vi "AI Timestamp Precision.vi"() -> ()   [LabVIEW 2020]
uses:
  <vilib>/DAQmx/read.llb/DAQmx Read (Analog Wfm 1Chan NSamp).vi
  <vilib>/DAQmx/write.llb/DAQmx Write (Digital Bool 1Line 1Point).vi
  <vilib>/Utility/High Resolution Relative Seconds.vi
  Utility VIs/Controls/Utilities-Wait.vi/89bc9713-8f2c-40bd-a11f-1c800a437687.vi
  <vilib>/DAQmx/create/channels.llb/DAQmx Create Channel (DO-Digital Output).vi
  <vilib>/DAQmx/create/channels.llb/DAQmx Create Channel (AI-Voltage-Basic).vi
  <vilib>/DAQmx/configure/timing.llb/DAQmx Timing (Sample Clock).vi
  <vilib>/DAQmx/miscellaneous.llb/DAQmx Fill In Error Info.vi
  <vilib>/Utility/High Resolution Polling Wait.vi
panel:
  out "Iteration":i32
  out "Graph":waveform(dbl)(graph)
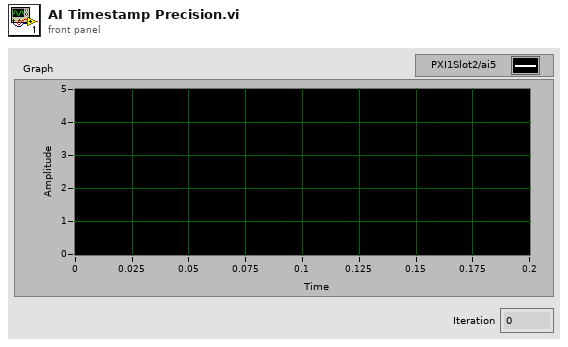
[diagram p1: front panel]
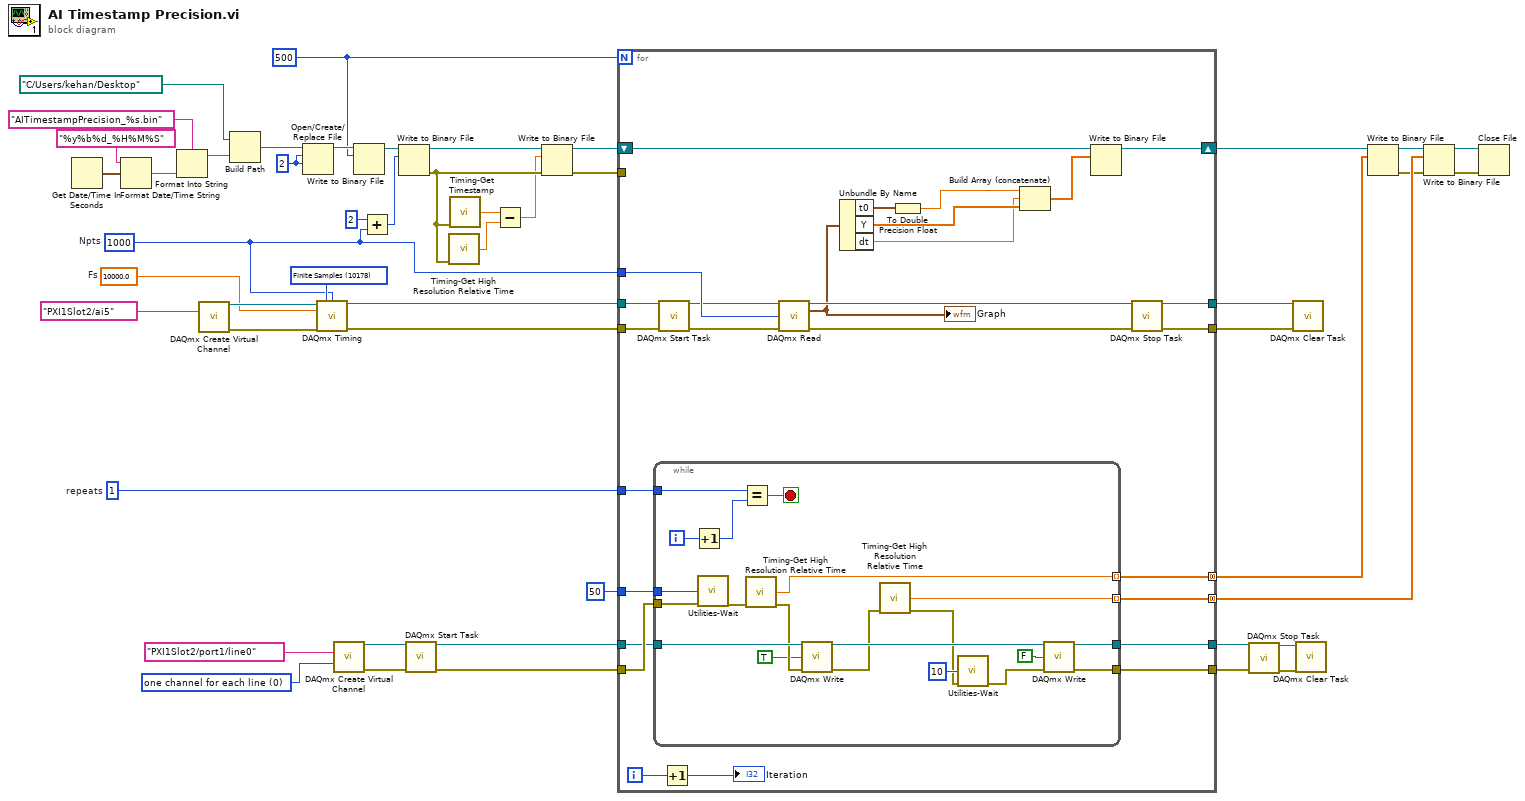
[diagram p0: block diagram]
diagram:
  w1 = 500
  w25 = u16 2
  w40 = 10000.0  # Fs
  w21 = 1000  # Npts
  w42 = 10178 items=["Finite Samples"=10178, "Continuous Samples"=10123, "Hardware Timed Single Point"=12522] ("sample mode")
  w22 = 1  # repeats
  w48 = 0 items=["one channel for each line", "one channel for all lines"] ("line grouping")
  n1 = Get Date/Time In Seconds() -> (seconds since 1Jan1904=w39:timestamp)
  n2 = Format Date/Time String(time format string (%c)="%y%b%d_%H%M%S", seconds (now)=w39) -> (date/time string=w37:string)  [unwired: 1 in]
  n3 = Format Into String(format string="AITimestampPrecision_%s.bin", w37) -> (resulting string=w34:string)  [unwired: 2 in, 1 out]
  n4 = call-poly <vilib>:"DAQmx Create Virtual Channel.vi"("physical channels"=tag "PXI1Slot2/ai5") -> ("task out"=w44:refnum<k21>, "error out"=w43:errorcluster)  [unwired: 13 in]
  n5 = Build Path(base path=path "C:/Users/kehan/Desktop" ("file path (use dialog)"), name or relative path=w34) -> (appended path=w33:path)
  n6 = Open/Create/Replace File(file path (use dialog)=w33, operation (0:open)=w25, access (0:read/write)=w25) -> (refnum out=w24:refnum<file>)  [unwired: 3 in, 2 out]
  n7 = call-poly <vilib>:"DAQmx Timing.vi"("task/channels in"=w44, "sample mode"=w42, "samples per channel"=w21, "rate"=w40, "error in"=w43) -> ("task out"=w11:refnum<k21>, "error out"=w10:errorcluster)  [unwired: 9 in]
  n8 = call-poly <vilib>:"DAQmx Create Virtual Channel.vi"("lines"=tag "PXI1Slot2/port1/line0", "line grouping"=w48) -> ("task out"=w46:refnum<k21>, "error out"=w45:errorcluster)  [unwired: 12 in]
  n9 = Write to Binary File(file (use dialog)=w24, data=w1) -> (refnum out=w23:refnum<file>)  [unwired: 4 in, 2 out]
  n10 = Add(x=2, y=w21) -> (x+y=w20:i32)
  n11 = Write to Binary File(file (use dialog)=w23, data=w20) -> (refnum out=w17:refnum<file>, error out=w16:errorcluster)  [unwired: 4 in, 1 out]
  n12 = call <vilib>:"DAQmx Start Task.vi"("task/channels in"=w46, "error in"=w45) -> ("task out"=w2:refnum<k21>, "error out"=w3:errorcluster)  [unwired: 12 in]
  n13 = call "Timing-Get High Resolution Relative Time.vi"("error in (no error)"=w16) -> ("double precision float"=w13:dbl)  [unwired: 13 in, 1 out]
  n14 = call "Timing-Get Timestamp.vi"("error in (no error)"=w16) -> ("double precision float"=w14:dbl)  [unwired: 13 in, 1 out]
  n15 = Subtract(x=w14, y=w13) -> (x-y=w12:dbl)
  n16 = Write to Binary File(file (use dialog)=w17, data=w12, error in=w16) -> (refnum out=w18:refnum<file>, error out=w15:errorcluster)  [unwired: 3 in, 1 out]
  n17 = for {
    N: w1 -> [_]
    tunnel: u32 50 ("milliseconds to wait") -> [w76]
    tunnel: [w71] -> w29 mode=concatenating
    tunnel: w22 -> [w70]
    tunnel: w21 -> [w69]
    tunnel: w15 -> [_]
    shift-right: [w73] -> w32
    shift-left: w18 -> [w68]
    tunnel: w11 -> [w61]
    tunnel: w10 -> [w60]
    tunnel: [w57] -> w9
    tunnel: [w56] -> w8
    tunnel: [w55] -> w7
    tunnel: [w54] -> w6
    tunnel: w3 -> [w53]
    tunnel: w2 -> [w52]
    tunnel: [w72] -> w31 mode=concatenating
    i -> [w51]
    n18 = while {
      tunnel: w52 -> [w96]
      tunnel: [w92] -> w55
      tunnel: [w91] -> w54
      tunnel: [w89] -> w71 mode=indexing
      tunnel: w70 -> [w90]
      tunnel: w76 -> [w88]
      tunnel: [w80] -> w72 mode=indexing
      tunnel: w53 -> [w77]
      i -> [w84]
      stop <- w85 stop-if-true
      n19 = Increment(x=w84) -> (x+1=w83:i32)
      n20 = call "Utilities-Wait.vi"("milliseconds to wait"=w88, "error in (no error)"=w77) -> ("error out"=w82:errorcluster)  [unwired: 13 in]
      n21 = Equal?(x=w90, y=w83) -> (x = y?=w85:bool)
      n22 = call "Timing-Get High Resolution Relative Time.vi"("error in (no error)"=w82) -> ("double precision float"=w80:dbl, "error out"=w81:errorcluster)  [unwired: 13 in]
      n23 = call-poly <vilib>:"DAQmx Write.vi"("task/channels in"=w96, "data"=TRUE, "error in"=w81) -> ("task out"=w94:refnum<k21>, "error out"=w87:errorcluster)  [unwired: 10 in, 1 out]
      n24 = call "Timing-Get High Resolution Relative Time.vi"("error in (no error)"=w87) -> ("double precision float"=w89:dbl, "error out"=w86:errorcluster)  [unwired: 13 in]
      n25 = call "Utilities-Wait.vi"("milliseconds to wait"=u32 10, "error in (no error)"=w86) -> ("error out"=w93:errorcluster)  [unwired: 13 in]
      n26 = call-poly <vilib>:"DAQmx Write.vi"("task/channels in"=w94, "data"=FALSE, "error in"=w93) -> ("task out"=w92:refnum<k21>, "error out"=w91:errorcluster)  [unwired: 10 in, 1 out]
    }
    n27 = call <vilib>:"DAQmx Start Task.vi"("task/channels in"=w61, "error in"=w60) -> ("task out"=w59:refnum<k21>, "error out"=w58:errorcluster)  [unwired: 12 in]
    n28 = Increment(x=w51) -> (x+1=→"Iteration":i32)
    n29 = call-poly <vilib>:"DAQmx Read.vi"("task/channels in"=w59, "number of samples per channel"=w69, "error in"=w58) -> ("task out"=w75:refnum<k21>, "data"=w67:waveform(dbl), "error out"=w74:errorcluster)  [unwired: 10 in]
    "Graph" <- w67
    n30 = Unbundle By Name(w67) -> ("t0"=w66:timestamp, "Y"=w63:dbl[], "dt"=w62:dbl)
    n31 = To Double Precision Float(number=w66) -> (double precision float=w65:dbl)
    n32 = Build Array (concatenate)(w65, w62, w63) -> (w64:dbl[])
    n33 = Write to Binary File(file (use dialog)=w68, data=w64) -> (refnum out=w73:refnum<file>)  [unwired: 4 in, 2 out]
    n34 = call <vilib>:"DAQmx Stop Task.vi"("task/channels in"=w75, "error in"=w74) -> ("task out"=w56:refnum<k21>, "error out"=w57:errorcluster)  [unwired: 12 in]
  }
  n35 = call <vilib>:"DAQmx Stop Task.vi"("task/channels in"=w7, "error in"=w6) -> ("task out"=w5:refnum<k21>, "error out"=w4:errorcluster)  [unwired: 12 in]
  n36 = call <vilib>:"DAQmx Clear Task.vi"("task in"=w8, "error in"=w9) -> ()  [unwired: 13 in, 1 out]
  n37 = call <vilib>:"DAQmx Clear Task.vi"("task in"=w5, "error in"=w4) -> ()  [unwired: 13 in, 1 out]
  n38 = Write to Binary File(file (use dialog)=w32, data=w31) -> (refnum out=w30:refnum<file>, error out=w26:errorcluster)  [unwired: 4 in, 1 out]
  n39 = Write to Binary File(file (use dialog)=w30, data=w29, error in=w26) -> (refnum out=w27:refnum<file>, error out=w28:errorcluster)  [unwired: 3 in, 1 out]
  n40 = Close File(refnum=w27, error in=w28) -> ()  [unwired: 2 out]
